vi "Get User Interface VI.vi"(8 "error in (no error)":errorcluster, 11 "Component Settings Editor in":refnum<class "Component Settings Editor.lvclass">) -> (0 "error out":errorcluster, 2 "user interface vi":refnum<vi>, 3 "Component Settings Editor out":refnum<class "Component Settings Editor.lvclass">)   [LabVIEW 2019, in "DSF Core.lvlib" / "Component Settings Editor.lvclass"]
uses:
  Component Settings Editor.lvclass
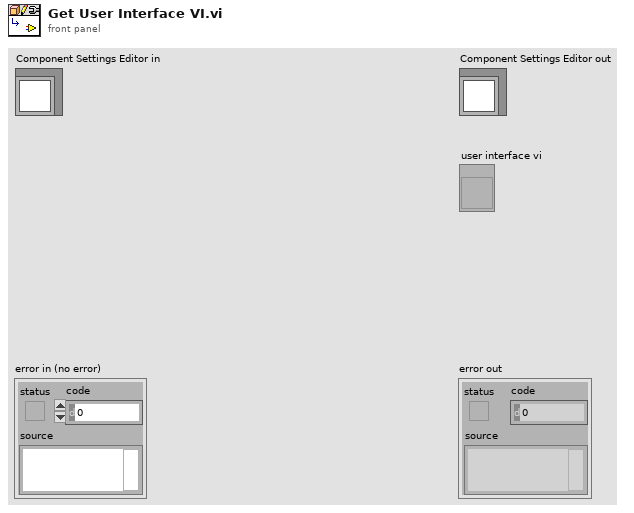
[diagram p1: front panel]
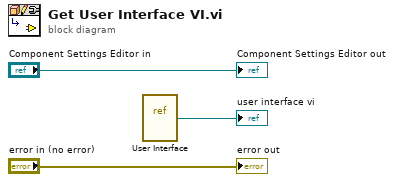
[diagram p0: block diagram]
diagram:
  n1 = vi-ref "User Interface.vi"() -> (→"user interface vi":refnum<vi>)
  "error out" <- "error in (no error)"
  "Component Settings Editor out" <- "Component Settings Editor in"
